vi "main.vi"() -> ()   [LabVIEW 2016]
uses:
  <vilib>/Platform/TimedLoop/XDataNode/timing_clust.ctl
  <vilib>/Platform/TimedLoop/XDataNode/nitl_modes.ctl
  <vilib>/Platform/TimedLoop/XDataNode/wakeup.ctl
  <vilib>/platform/TimedLoop/XDataNode/XDataNode.xnode
  <vilib>/Platform/TimedLoop/XDataNode/XDNodeRunTimeDep.lvlib
  <instrlib>/Lake Shore 425/Lake Shore 425.lvlib
panel:
  out "duration":dbl
  in  "Measure":bool
  out "z [mm]":dbl
  out "y [mm]":dbl
  out "x [mm]":dbl
  in  "z":dbl caption="z [mm]"
  in  "y":dbl caption="y [mm]"
  in  "x":dbl caption="x [mm]"
  in  "Map Mode":bool
  in  "Position File":path=path "C:/Users/ephenix/git/LabViewVIs/MegaVIEW/LabVIEW_tests/position_file_loading/position test.txt"
  out "XY Graph":cluster{dbl[], dbl[]}[](graph)
  in  "Y-Axis":i32(ring)=6 items=["Time"=0, "x position"=1, "y position"=2, "z position"=3, "Gaussmeter 1"=4, "Gaussmeter 2"=6, "Gaussmeter 3"=8, "Multimeter"=10, "Temperature 1"=11, "Temperature 2"=12, "Temperature 3"=13, "Temperature 4"=14, "Temperature 5"=15, "Temperature 6"=16, "Temperature 7"=17, "Temperature 8"=18]
  in  "X-Axis":i32(ring)=4 items=["Time"=0, "x position"=1, "y position"=2, "z position"=3, "Gaussmeter 1"=4, "Gaussmeter 2"=6, "Gaussmeter 3"=8, "Multimeter"=10, "Temperature 1"=11, "Temperature 2"=12, "Temperature 3"=13, "Temperature 4"=14, "Temperature 5"=15, "Temperature 6"=16, "Temperature 7"=17, "Temperature 8"=18]
  in  "Period [s]":dbl=1.0
  in  "Seconds":dbl
  in  "Minutes":dbl
  in  "Hours":dbl
  in  "Moving Gaussmeter 3":bool caption="Moving"
  in  "x Gaussmeter 3":dbl caption="x [mm]"
  in  "y Gaussmeter 3":dbl caption="y [mm]"
  in  "z Gaussmeter 3":dbl caption="z [mm]"
  in  "Moving Gaussmeter 2":bool caption="Moving"
  in  "x Gaussmeter 2":dbl caption="x [mm]"
  in  "y Gaussmeter 2":dbl caption="y [mm]"
  in  "z Gaussmeter 2":dbl caption="z [mm]"
  in  "z Gaussmeter 1":dbl caption="z [mm]"
  in  "y Gaussmeter 1":dbl caption="y [mm]"
  in  "x Gaussmeter 1":dbl caption="x [mm]"
  in  "Moving Gaussmeter 1":bool caption="Moving"
  out "Time [s]":dbl
  in  "Stop Button":bool
  out "Output File Name":string
  out "Output File Path":path
  in  "Output Folder Path":path=path "C:/Users/ephenix/Dropbox/Stony Brook Research Team Folder/LabVIEW/VI_Argonne/MegaVIEW_v_0_0_5/test output"
  in  "Switch Gaussmeter 3":bool
  in  "VISA resource name Gaussmeter 3":refnum<visa-resource-name>
  out "Probe Type 3":u16(ring)=40 caption="Probe Type" items=["High Sensitivity"=40, "High Stability"=41, "Ultra-High Sensitivity"=42, "User Programmable Cable / High Sensitivity Probe"=50, "User Programmable Cable / High Stability Probe"=51, "User Programmable Cable / Ultra-High Sensitivity Probe"=52]
  out "Probe Serial Number 3":string caption="Probe Serial Number"
  out "Probe Sensitivity 3":dbl=0.001 caption="Probe Sensitivity" format="%^.3e"
  out "Field\nComp 3":bool caption="Field\nComp"
  out "Field Range  3":u16(ring)=1 caption="Field Range" items=["1 - Lowest"=1, "2"=2, "3"=3, "4 - Highest"=4]
  out "Field Units 3":u16(ring)=1 caption="Field Units" items=["Gauss"=1, "Tesla"=2, "Oersted"=3, "Amp/Meter"=4]
  out "Auto\nRange 3":bool caption="Auto\nRange"
  out "Status Gaussmeter 3":bool caption="Status"
  in  "Switch Gaussmeter 2":bool
  in  "VISA resource name Gaussmeter 2":refnum<visa-resource-name>
  out "Probe Type 2":u16(ring)=40 caption="Probe Type" items=["High Sensitivity"=40, "High Stability"=41, "Ultra-High Sensitivity"=42, "User Programmable Cable / High Sensitivity Probe"=50, "User Programmable Cable / High Stability Probe"=51, "User Programmable Cable / Ultra-High Sensitivity Probe"=52]
  out "Probe Serial Number 2":string caption="Probe Serial Number"
  out "Probe Sensitivity 2":dbl=0.001 caption="Probe Sensitivity" format="%^.3e"
  out "Field\nComp 2":bool caption="Field\nComp"
  out "Field Range  2":u16(ring)=1 caption="Field Range" items=["1 - Lowest"=1, "2"=2, "3"=3, "4 - Highest"=4]
  out "Field Units 2":u16(ring)=1 caption="Field Units" items=["Gauss"=1, "Tesla"=2, "Oersted"=3, "Amp/Meter"=4]
  out "Auto\nRange 2":bool caption="Auto\nRange"
  out "Status Gaussmeter 2":bool caption="Status"
  out "Status Gaussmeter 1":bool caption="Status"
  out "Auto\nRange":bool
  out "Field Units":u16(ring)=1 items=["Gauss"=1, "Tesla"=2, "Oersted"=3, "Amp/Meter"=4]
  out "Field Range":u16(ring)=1 items=["1 - Lowest"=1, "2"=2, "3"=3, "4 - Highest"=4]
  out "Field\nComp":bool
  out "Probe Sensitivity":dbl=0.001 format="%^.3e"
  out "Probe Serial Number":string
  out "Probe Type":u16(ring)=40 items=["High Sensitivity"=40, "High Stability"=41, "Ultra-High Sensitivity"=42, "User Programmable Cable / High Sensitivity Probe"=50, "User Programmable Cable / High Stability Probe"=51, "User Programmable Cable / Ultra-High Sensitivity Probe"=52]
  in  "VISA resource name Temperature Monitor":refnum<visa-resource-name>
  in  "VISA resource name Multimeter":refnum<visa-resource-name>
  in  "VISA resource name Gaussmeter 1":refnum<visa-resource-name>
  in  "Switch Temperature Monitor":bool
  in  "Switch Multimeter":bool
  in  "Switch Gaussmeter 1":bool
  out "Waveform Chart Temperature Monitor":dbl(graph)
  out "Waveform Chart Multimeter":dbl(graph)
  out "Waveform Chart Gaussmeter 3":dbl(graph)
  out "Waveform Chart Gaussmeter 2":dbl(graph)
  out "Waveform Chart Gaussmeter 1":dbl(graph)
  # "Gaussmeter 1 (Lake Shore 425)"
  # "Gaussmeter 2 (Lake Shore 425)"
  # "Gaussmeter 3 (Lake Shore 425)"
  # "Multimeter (Agilent 34461A)"
  # "Temperature Monitor (Lake Shore 218)"
  # "XY Graph Axes"
  # "Duration"
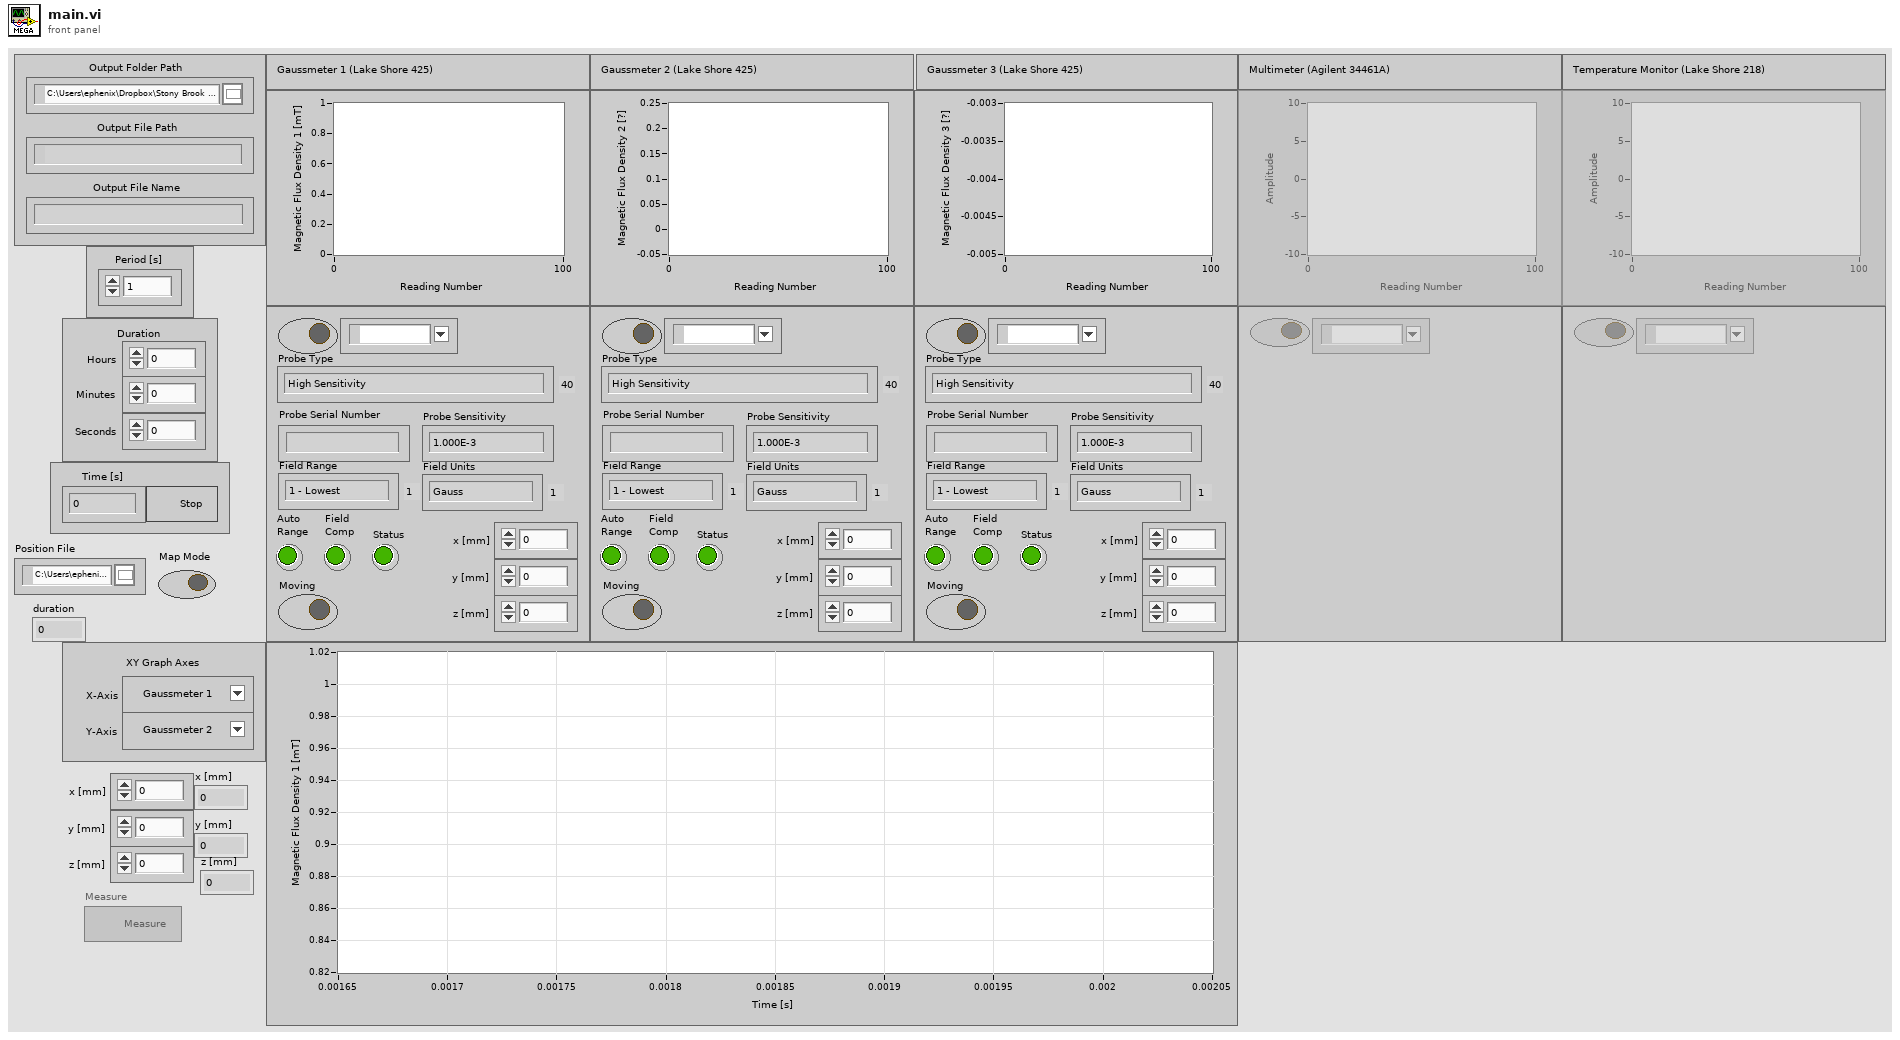
[diagram p1: front panel]
types:
  T1 = cluster{"Gaussmeter VISA resource name out":refnum<visa-resource-name>, "Switch Gaussmeter 1":bool, "Gaussmeter VISA resource name out":refnum<visa-resource-name>, "Switch Gaussmeter 2":bool, "Gaussmeter VISA resource name out":refnum<visa-resource-name>, "Switch Gaussmeter 3":bool}
  T2 = enum16{"open", "replace", "create", "open or create", "replace or create", "replace or create with confirmation"}
  T3 = enum8{"Enabled", "Disabled", "Disabled and Grayed Out"}
  T4 = typedef "XDNodeRunTimeDep.lvlib/timing_clust.ctl" = cluster{"Expected End [f-1]":u64, "Actual End [f-1]":u64, "Finished Late? [f-1]":bool, "Expected End [i-1]":u64, "Actual End [i-1]":u64, "Finished Late? [i-1]":bool, "Expected Start [i]":u64, "Actual Start [i]":u64, "Expected Start [f]":u64, "Actual Start [f]":u64, "Source Name":string, "Structure Name":string, "Period":i64, "Deadline":i64, "Offset":i64, "Start":i64, "Priority":i32, "Timeout":i32, "Mode":T5, "Wakeup Reason":T6, "Error":errorcluster, "Source Type":string, "Secondary Source Type":string, "Global End Time":u64, "Global Start Time":u64, "Frame Duration":u64, "Iteration Duration":u64, "Assigned CPU":i32, "I/O Scan Engine Mode":u32}
  T5 = typedef "XDNodeRunTimeDep.lvlib/nitl_modes.ctl" = enum32{"No Change", "Process missed periods, maintain original phase", "Discard missed periods, maintain original phase", "Process missed periods, ignore original phase", "Discard missed periods, ignore original phase"}
  T6 = typedef "XDNodeRunTimeDep.lvlib/wakeup.ctl" = enum32{"Normal", "Aborted", "Asynchronous wakeup", "Timing source error", "Timed loop error", "Timeout"}
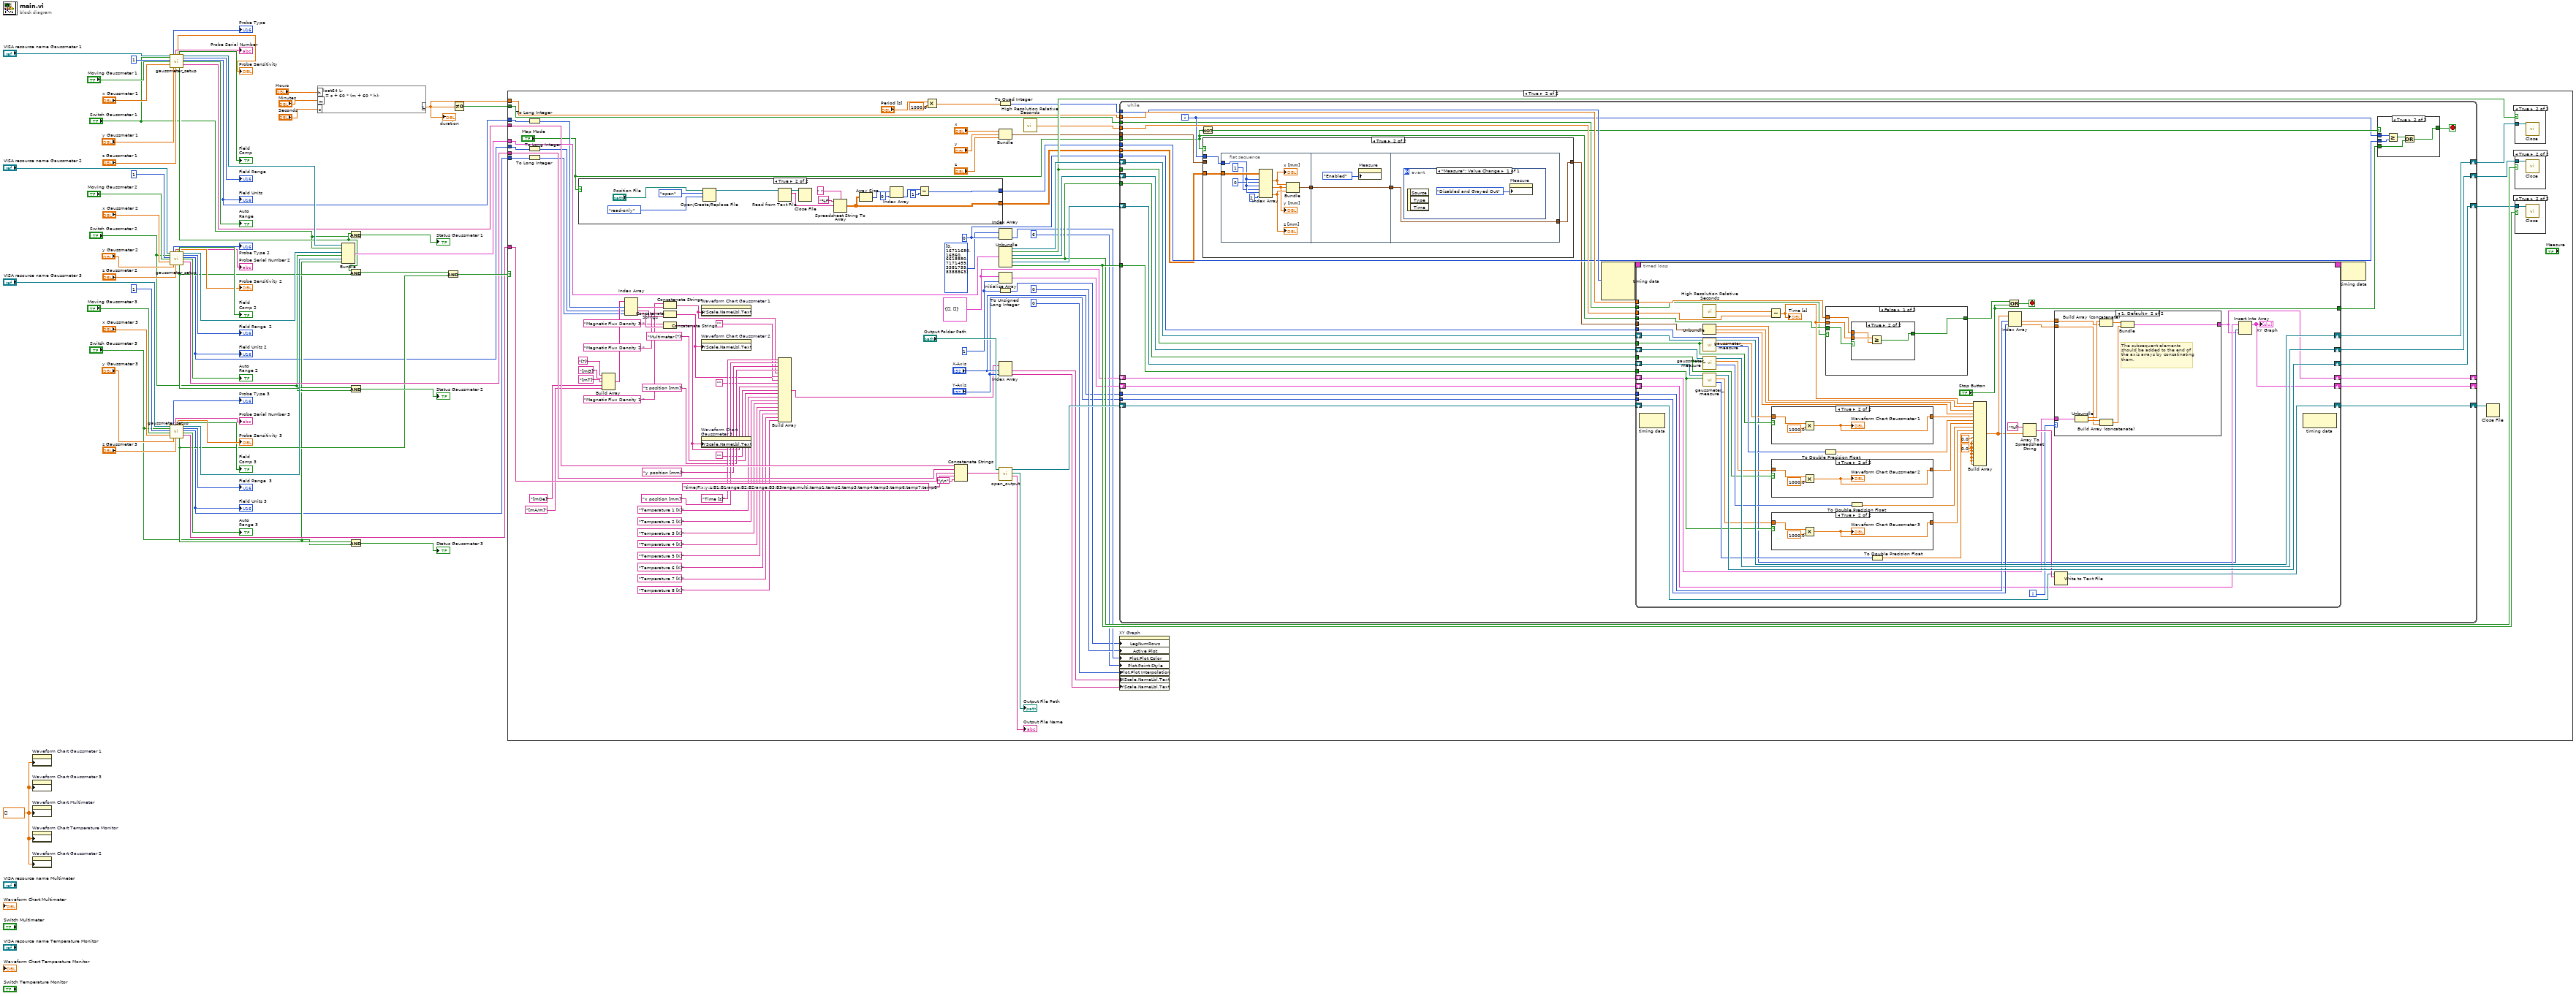
[diagram p0: block diagram]
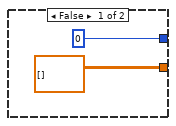
[diagram p3: hidden frame]
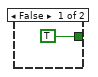
[diagram p5: hidden frame]
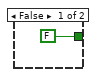
[diagram p6: hidden frame]
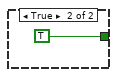
[diagram p7: hidden frame]
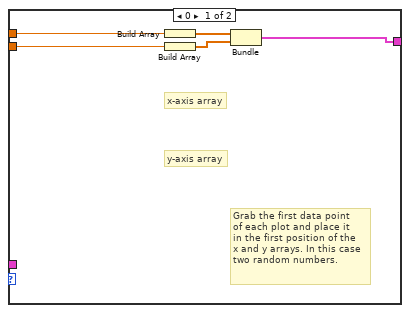
[diagram p8: hidden frame]
diagram:
  w8 = dbl[] [] ("History Data")
  n1 = property on="Waveform Chart Gaussmeter 1" class="WFChart (strict)"("History Data"=w8) -> ()  [unwired: 2 in, 2 out]
  n2 = property on="Waveform Chart Gaussmeter 3" class="WFChart (strict)"("History Data"=w8) -> ()  [unwired: 2 in, 2 out]
  n3 = property on="Waveform Chart Multimeter" class="WFChart (strict)"("History Data"=w8) -> ()  [unwired: 2 in, 2 out]
  n4 = property on="Waveform Chart Temperature Monitor" class="WFChart (strict)"("History Data"=w8) -> ()  [unwired: 2 in, 2 out]
  n5 = property on="Waveform Chart Gaussmeter 2" class="WFChart (strict)"("History Data"=w8) -> ()  [unwired: 2 in, 2 out]
  n6 = call "gaussmeter_setup.vi"("VISA resource name Gaussmeter"="VISA resource name Gaussmeter 1", "Switch Gaussmeter"="Switch Gaussmeter 1", "Gaussmeter Number"=u8 1, "Moving Gaussmeter"="Moving Gaussmeter 1", "x Gaussmeter"="x Gaussmeter 1", "y Gaussmeter"="y Gaussmeter 1", "z Gaussmeter"="z Gaussmeter 1") -> ("Probe Type"=→"Probe Type":u16, "Probe Serial Number"=→"Probe Serial Number":string, "Probe Sensitivity"=→"Probe Sensitivity":dbl, "Probe Field\nCompensation On"=→"Field\nComp":bool, "Status Gaussmeter"=w16:bool, "Gaussmeter VISA resource name out"=w40:refnum<visa-resource-name>, "Field Range"=→"Field Range":u16, "Field Units"=w5:u16, "Auto Range On"=→"Auto\nRange":bool, "Text Output"=w34:string)  [unwired: 2 in, 1 out]
  "Field Units" <- w5
  n7 = call "gaussmeter_setup.vi"("VISA resource name Gaussmeter"="VISA resource name Gaussmeter 2", "Switch Gaussmeter"="Switch Gaussmeter 2", "Gaussmeter Number"=u8 1, "Moving Gaussmeter"="Moving Gaussmeter 2", "x Gaussmeter"="x Gaussmeter 2", "y Gaussmeter"="y Gaussmeter 2", "z Gaussmeter"="z Gaussmeter 2") -> ("Probe Type"=→"Probe Type 2":u16, "Probe Serial Number"=→"Probe Serial Number 2":string, "Probe Sensitivity"=→"Probe Sensitivity 2":dbl, "Probe Field\nCompensation On"=→"Field\nComp 2":bool, "Status Gaussmeter"=w13:bool, "Gaussmeter VISA resource name out"=w39:refnum<visa-resource-name>, "Field Range"=→"Field Range  2":u16, "Field Units"=w6:u16, "Auto Range On"=→"Auto\nRange 2":bool, "Text Output"=w33:string)  [unwired: 2 in, 1 out]
  "Field Units 2" <- w6
  n8 = call "gaussmeter_setup.vi"("VISA resource name Gaussmeter"="VISA resource name Gaussmeter 3", "Switch Gaussmeter"="Switch Gaussmeter 3", "Gaussmeter Number"=u8 1, "Moving Gaussmeter"="Moving Gaussmeter 3", "x Gaussmeter"="x Gaussmeter 3", "y Gaussmeter"="y Gaussmeter 3", "z Gaussmeter"="z Gaussmeter 3") -> ("Probe Type"=→"Probe Type 3":u16, "Probe Serial Number"=→"Probe Serial Number 3":string, "Probe Sensitivity"=→"Probe Sensitivity 3":dbl, "Probe Field\nCompensation On"=→"Field\nComp 3":bool, "Status Gaussmeter"=w11:bool, "Gaussmeter VISA resource name out"=w38:refnum<visa-resource-name>, "Field Range"=→"Field Range  3":u16, "Field Units"=w7:u16, "Auto Range On"=→"Auto\nRange 3":bool, "Text Output"=w32:string)  [unwired: 2 in, 1 out]
  "Field Units 3" <- w7
  n9 = formula code="float64 L;\nL = s + 60 * (m + 60 * h);"("h"="Hours", "m"="Minutes", "s"="Seconds") -> ("L"=w1:dbl)
  "duration" <- w1
  n10 = Bundle("Gaussmeter VISA resource name out"=w40, "Switch Gaussmeter 1"="Switch Gaussmeter 1", "Gaussmeter VISA resource name out"=w39, "Switch Gaussmeter 2"="Switch Gaussmeter 2", "Gaussmeter VISA resource name out"=w38, "Switch Gaussmeter 3"="Switch Gaussmeter 3") -> (w35:T1)  [unwired: 1 in]
  n11 = And(x=w16, y="Switch Gaussmeter 1") -> (x .and. y?=→"Status Gaussmeter 1":bool)
  n12 = And(x=w16, y=w13) -> (x .and. y?=w37:bool)
  n13 = And(x=w13, y="Switch Gaussmeter 2") -> (x .and. y?=→"Status Gaussmeter 2":bool)
  n14 = And(x=w11, y="Switch Gaussmeter 3") -> (x .and. y?=→"Status Gaussmeter 3":bool)
  n15 = And(x=w37, y=w11) -> (x .and. y?=w36:bool)
  n16 = Not Equal To 0?(x=w1) -> (x != 0?=w18:bool)
  n17 = case shown="True" w36 {
    tunnel: w35 -> [_ w150]
    tunnel: w34 -> [_ w142]
    tunnel: w33 -> [_ w141]
    tunnel: w32 -> [_ w140]
    tunnel: w18 -> [_ w128]
    tunnel: w1 -> [_ w127]
    tunnel: w7 -> [_ w82]
    tunnel: w6 -> [_ w81]
    tunnel: w5 -> [_ w80]
    frame False {
    }
    frame True {
      w120 = 0
      w113 = 1 ("dimension size")
      w122 = cluster{dbl[], dbl[]} {[], []}
      n18 = To Long Integer(number=w80) -> (32bit integer=w86:i32)
      n19 = To Long Integer(number=w81) -> (32bit integer=w84:i32)
      n20 = To Long Integer(number=w82) -> (32bit integer=w83:i32)
      n21 = case shown="True" "Map Mode" {
        tunnel: [0 w154] -> w69
        tunnel: [dbl[][] [] w153] -> w68
        frame False {
        }
        frame True {
          n22 = Open/Create/Replace File(file path (use dialog)="Position File", operation (0:open)=T2."open", access (0:read/write)=enum16{"read/write", "read-only", "write-only"}."read-only") -> (refnum out=w164:refnum<file>)  [unwired: 3 in, 2 out]
          n23 = Read from Text File(file (use dialog)=w164) -> (refnum out=w163:refnum<file>, text=w162:string)  [unwired: 3 in, 2 out]
          n24 = Close File(refnum=w163) -> ()  [unwired: 1 in, 2 out]
          n25 = Spreadsheet String To Array(delimiter (Tab)=" ", format string="%f", spreadsheet string=w162) -> (array=w153:dbl[][])  [unwired: 1 in]
          n26 = Array Size(array=w153) -> (size(s)=w158:i32[])
          n27 = Index Array(array=w158, index=0) -> (element=w156:i32)
          n28 = Subtract(x=w156, y=1) -> (x-y=w154:i32)
        }
      }
      n29 = Build Array("[?]", "[mG]", "[mT]", "[mOe]", "[mA/m]") -> (w85:string[])
      n30 = Index Array(array=w85, index #1=w86, index #2=w84, index #3=w83) -> (element #1=w77:string, element #2=w78:string, element #3=w79:string)
      n31 = Concatenate Strings("Magnetic Flux Density 1 ", w77) -> (w71:string)
      n32 = Concatenate Strings("Magnetic Flux Density 2 ", w78) -> (w72:string)
      n33 = Concatenate Strings("Magnetic Flux Density 3 ", w79) -> (w73:string)
      n34 = property on="Waveform Chart Gaussmeter 1" class="WFChart (strict)"("YScale.NameLbl.Text"=w71) -> ()  [unwired: 2 in, 2 out]
      n35 = property on="Waveform Chart Gaussmeter 2" class="WFChart (strict)"("YScale.NameLbl.Text"=w72) -> ()  [unwired: 2 in, 2 out]
      n36 = property on="Waveform Chart Gaussmeter 3" class="WFChart (strict)"("YScale.NameLbl.Text"=w73) -> ()  [unwired: 2 in, 2 out]
      n37 = Build Array("Time [s]", "x position [mm]", "y position [mm]", "z position [mm]", w71, "", w72, "", w73, "", "Multimeter [?]", "Temperature 1 [K]", "Temperature 2 [K]", "Temperature 3 [K]", "Temperature 4 [K]", "Temperature 5 [K]", "Temperature 6 [K]", "Temperature 7 [K]", "Temperature 8 [K]") -> (w106:string[])
      n38 = Multiply(x="Period [s]", y=1000.0) -> (x*y=w123:dbl)
      n39 = Concatenate Strings(w142, w141, w140, "time/F:x:y:z:B1:B1range:B2:B2range:B3:B3range:multi:temp1:temp2:temp3:temp4:temp5:temp6:temp7:temp8", "\r\n") -> (w143:string)
      n40 = To Quad Integer(1:w123) -> (0:w126:i64)
      n41 = To Unsigned Long Integer(number=w113) -> (unsigned 32bit integer=w114:u32)
      n42 = Bundle("x"="x", "y"="y", "z"="z") -> (w64:cluster{"x":dbl, "y":dbl, "z":dbl})  [unwired: 1 in]
      n43 = Index Array(array=u32[] [0, 16711680, 16860, 6618880, 7171459, 3381759, 8388863], index=w120) -> (element=w118:u32)
      n44 = Unbundle(w150) -> ("Gaussmeter VISA resource name out"=w149:refnum<visa-resource-name>, "Switch Gaussmeter 1"=w133:bool, "Gaussmeter VISA resource name out"=w148:refnum<visa-resource-name>, "Switch Gaussmeter 2"=w134:bool, "Gaussmeter VISA resource name out"=w147:refnum<visa-resource-name>, "Switch Gaussmeter 3"=w135:bool)
      n45 = Initialize Array(w122, w113) -> (w121:cluster{dbl[], dbl[]}[])
      n46 = Index Array(array=w106, index #1="X-Axis", index #2="Y-Axis") -> (element #1=w105:string, element #2=w104:string)
      n47 = call "open_output.vi"("Output File Header"=w143, "Output Folder Path"="Output Folder Path") -> ("Output File Name"=→"Output File Name":string, "Output File Path"=→"Output File Path":path, "refnum out"=w137:refnum<file>)  [unwired: 7 in]
      n48 = call <vilib>:"High Resolution Relative Seconds.vi"() -> ("relative seconds"=w129:dbl)
      n49 = while {
        tunnel: w135 -> [w192]
        tunnel: w134 -> [w191]
        tunnel: w133 -> [w190]
        tunnel: w129 -> [w186]
        tunnel: w128 -> [w169]
        tunnel: w127 -> [w185]
        tunnel: w126 -> [w184]
        tunnel: w120 -> [w181]
        tunnel: "X-Axis" -> [w180]
        tunnel: "Y-Axis" -> [w179]
        tunnel: "Map Mode" -> [w171]
        shift-right: [w189] -> w132
        shift-left: w149 -> [w197]
        shift-right: [w188] -> w131
        shift-left: w148 -> [w196]
        shift-right: [w187] -> w130
        shift-left: w147 -> [w195]
        shift-right: [w193] -> w136
        shift-left: w137 -> [w194]
        tunnel: w69 -> [w176]
        tunnel: w68 -> [w170]
        tunnel: w64 -> [w173]
        shift-right: [w168] -> _
        shift-left: w122 -> [w183]
        shift-right: [w167] -> _
        shift-left: w121 -> [w182]
        i -> [w172]
        stop <- w177 stop-if-true
        n50 = Not(x=w171) -> (.not. x?=w175:bool)
        n51 = case shown="True" w171 {
          tunnel: w170 -> [_ w205]
          tunnel: [w200 w204] -> w174
          tunnel: w173 -> [w200 _]
          tunnel: w172 -> [_ w203]
          frame False {
          }
          frame True {
            n52 = flat-sequence {
              tunnel: w205 -> [w214]
              tunnel: w203 -> [w209]
              tunnel: [w213] -> w202
              tunnel: w202 -> [w216]
              tunnel: [w216] -> w201
              tunnel: [w217] -> w204
              tunnel: w201 -> [w217]
              frame #0 {
                n53 = Index Array(array=w214, index (row) #1=w209, index (col) #1=0 ("disabled index (col)"), index (row) #2=w209, index (col) #2=1 ("disabled index (col)"), index (row) #3=w209, index (col) #3=2 ("disabled index (col)")) -> (element #1=w210:dbl, element #2=w211:dbl, element #3=w212:dbl)
                "x [mm]" <- w210
                "y [mm]" <- w211
                "z [mm]" <- w212
                n54 = Bundle(w210, w211, w212) -> (w213:cluster{dbl, dbl, dbl})  [unwired: 1 in]
              }
              frame #1 {
                n55 = property on="Measure" class="Bool"("DisabledEnum"=T3."Enabled" ("Disabled")) -> ()  [unwired: 2 in, 2 out]
              }
              frame #2 {
                n56 = event shown="[0] \"Measure\": Value Change" {
                  selector: _ -> [_]
                  dyn-events: _ -> [_]
                  timeout: _ -> [_]
                  event "Measure": Value Change {
                    n57 = event-data() -> ()  [unwired: 1 in, 3 out]
                    n58 = property on="Measure" class="Bool"("DisabledEnum"=T3."Disabled and Grayed Out" ("Disabled")) -> ()  [unwired: 2 in, 2 out]
                  }
                }
              }
            }
          }
        }
        n59 = node-c288(w184) -> (w199:T4)  [unwired: 3 in]
        n60 = timed-loop {
          timing: w199 -> [_]
          timing-out: [_] -> w198
          shift-right: [w270] -> w189
          shift-left: w197 -> [w275]
          tunnel: w190 -> [w252]
          shift-right: [w271] -> w188
          shift-left: w196 -> [w274]
          shift-right: [w272] -> w187
          shift-left: w195 -> [w273]
          tunnel: w191 -> [w251]
          tunnel: w192 -> [w250]
          shift-right: [w261] -> w193
          shift-left: w194 -> [w262]
          tunnel: w186 -> [w256]
          tunnel: w185 -> [w229]
          tunnel: w180 -> [w249]
          tunnel: w179 -> [w248]
          shift-right: [w240] -> w168
          shift-left: w183 -> [w243]
          shift-right: [w239] -> w167
          shift-left: w182 -> [w242]
          tunnel: w181 -> [w241]
          tunnel: w171 -> [w227]
          tunnel: ["Stop Button"] -> w178
          tunnel: w174 -> [w230]
          tunnel: w169 -> [w226]
          i -> [w246]
          stop <- w255 stop-if-true
          w259 = 0.0
          n61 = node-c288() -> ()  [unwired: 1 in, 1 out]
          n62 = call <vilib>:"High Resolution Relative Seconds.vi"() -> ("relative seconds"=w257:dbl)
          n63 = Unbundle(w230) -> ("x"=w233:dbl, "y"=w232:dbl, "z"=w231:dbl)
          n64 = call "gaussmeter_measure.vi"("Switch Gaussmeter"=w252, "VISA resource name"=w275) -> ("Field Range"=w268:u16, "Field Reading"=w254:dbl, "VISA resource name out"=w270:refnum<visa-resource-name>)  [unwired: 5 in, 2 out]
          n65 = call "gaussmeter_measure.vi"("Switch Gaussmeter"=w251, "VISA resource name"=w274) -> ("Field Range"=w267:u16, "Field Reading"=w253:dbl, "VISA resource name out"=w271:refnum<visa-resource-name>)  [unwired: 5 in, 2 out]
          n66 = call "gaussmeter_measure.vi"("Switch Gaussmeter"=w250, "VISA resource name"=w273) -> ("Field Range"=w266:u16, "Field Reading"=w236:dbl, "VISA resource name out"=w272:refnum<visa-resource-name>)  [unwired: 5 in, 2 out]
          n67 = Subtract(x=w257, y=w256) -> (x-y=w228:dbl)
          "Time [s]" <- w228
          n68 = case shown="True" w252 {
            tunnel: w254 -> [w306 w308]
            tunnel: [w306 w307] -> w238
            frame False {
            }
            frame True {
              n69 = Multiply(x=w308, y=1000.0) -> (x*y=w307:dbl)
              "Waveform Chart Gaussmeter 1" <- w307
            }
          }
          n70 = case shown="True" w251 {
            tunnel: w253 -> [w302 w304]
            tunnel: [w302 w303] -> w235
            frame False {
            }
            frame True {
              n71 = Multiply(x=w304, y=1000.0) -> (x*y=w303:dbl)
              "Waveform Chart Gaussmeter 2" <- w303
            }
          }
          n72 = case shown="True" w250 {
            tunnel: w236 -> [w298 w300]
            tunnel: [w298 w299] -> w237
            frame False {
            }
            frame True {
              n73 = Multiply(x=w300, y=1000.0) -> (x*y=w299:dbl)
              "Waveform Chart Gaussmeter 3" <- w299
            }
          }
          n74 = To Double Precision Float(number=w268) -> (double precision float=w269:dbl)
          n75 = case shown="False" w226 {
            tunnel: w229 -> [w278 _]
            tunnel: w228 -> [w277 _]
            tunnel: w227 -> [w276 _]
            tunnel: [w279 TRUE] -> w225
            frame False {
              n76 = case shown="True" w276 {
                tunnel: w277 -> [_ w283]
                tunnel: w278 -> [_ w282]
                tunnel: [FALSE w281] -> w279
                frame False {
                }
                frame True {
                  n77 = Greater Or Equal?(x=w283, y=w282) -> (x >= y?=w281:bool)
                }
              }
            }
            frame True {
            }
          }
          n78 = To Double Precision Float(number=w267) -> (double precision float=w265:dbl)
          n79 = To Double Precision Float(number=w266) -> (double precision float=w264:dbl)
          n80 = Build Array(w228, w233, w232, w231, w238, w269, w235, w265, w237, w264, 0.0, w259, w259, w259, w259, w259, w259, w259, w259) -> (w247:dbl[])
          n81 = Or(x=w225, y="Stop Button") -> (x .or. y?=w255:bool)
          n82 = Index Array(array=w247, index #1=w249, index #2=w248) -> (element #1=w245:dbl, element #2=w244:dbl)
          n83 = Array To Spreadsheet String(array=w247, 3:"%f" ("format string")) -> (spreadsheet string=w263:string)  [unwired: 1 in]
          n84 = case shown="1, Default" w246 {
            tunnel: [w287 w294] -> w240
            tunnel: w243 -> [_ w290]
            tunnel: w244 -> [w285 w292]
            tunnel: w245 -> [w286 w291]
            frame 0 {
              # "y-axis array"
              # "x-axis array"
              # "Grab the first data point\nof each plot and place it\nin the first position of the \nx and y arrays. In this case\ntwo random numbers."
              n85 = Build Array(w286) -> (w289:dbl[])
              n86 = Build Array(w285) -> (w288:dbl[])
              n87 = Bundle(w289, w288) -> (w287:cluster{dbl[], dbl[]})  [unwired: 1 in]
            }
            frame 1, Default {
              # "The subsequent elements\nshould be added to the end of\nthe axis arrays by concatinating\nthem."
              n88 = Unbundle(w290) -> (w297:dbl[], w293:dbl[])
              n89 = Build Array (concatenate)(w297, w291) -> (w296:dbl[])
              n90 = Build Array (concatenate)(w293, w292) -> (w295:dbl[])
              n91 = Bundle(w296, w295) -> (w294:cluster{dbl[], dbl[]})  [unwired: 1 in]
            }
          }
          n92 = Write to Text File(file (use dialog)=w262, text=w263) -> (refnum out=w261:refnum<file>)  [unwired: 2 in, 2 out]
          n93 = Insert Into Array(array=w242, index=w241, new element=w240) -> (w239:cluster{dbl[], dbl[]}[])
          "XY Graph" <- w239
          n94 = node-c288() -> ()  [unwired: 1 in, 1 out]
        }
        n95 = node-c288(w198) -> ()  [unwired: 1 out]
        n96 = case shown="True" w175 {
          tunnel: w178 -> [_ w224]
          tunnel: [TRUE w223] -> w177
          tunnel: w176 -> [_ w222]
          tunnel: w172 -> [_ w221]
          frame False {
          }
          frame True {
            n97 = Greater Or Equal?(x=w221, y=w222) -> (x >= y?=w220:bool)
            n98 = Or(x=w220, y=w224) -> (x .or. y?=w223:bool)
          }
        }
      }
      n99 = property on="XY Graph" class="XYGraph (strict)"("LegNumRows"=w114, "Active Plot"=u32 0, "Plot.Plot Color"=w118, "Plot.Point Style"=u8 6, "Plot.Plot Interpolation"=u8 0, "XScale.NameLbl.Text"=w105, "YScale.NameLbl.Text"=w104) -> ()  [unwired: 2 in, 2 out]
      n100 = Close File(refnum=w136) -> ()  [unwired: 1 in, 2 out]
      n101 = case shown="True" w133 {
        tunnel: w132 -> [_ w318]
        frame False {
        }
        frame True {
          n102 = call <instrlib>:"Close.vi"("VISA resource name"=w318) -> ()  [unwired: 10 in, 1 out]
        }
      }
      n103 = case shown="True" w134 {
        tunnel: w131 -> [_ w317]
        frame False {
        }
        frame True {
          n104 = call <instrlib>:"Close.vi"("VISA resource name"=w317) -> ()  [unwired: 10 in, 1 out]
        }
      }
      n105 = case shown="True" w135 {
        tunnel: w130 -> [_ w316]
        frame False {
        }
        frame True {
          n106 = call <instrlib>:"Close.vi"("VISA resource name"=w316) -> ()  [unwired: 10 in, 1 out]
        }
      }
    }
  }
